vi "Zero.vi"(8 "error in (no error)":errorcluster, 11 "Simple Actor in":refnum<class "Simple Actor.lvclass">) -> (0 "error out":errorcluster, 3 "Simple Actor out":refnum<class "Simple Actor.lvclass">)   [LabVIEW 2012, in "Simple Actor.lvclass"]
uses:
  Simple Actor.lvclass
  Simple Actor.lvclass/Simple Actor.ctl
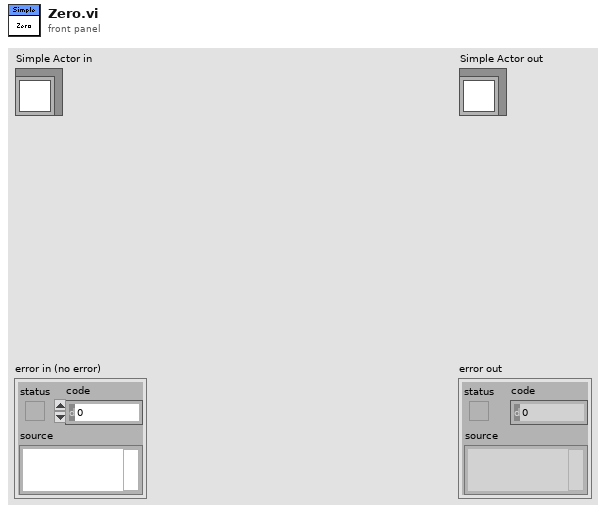
[diagram p1: front panel]
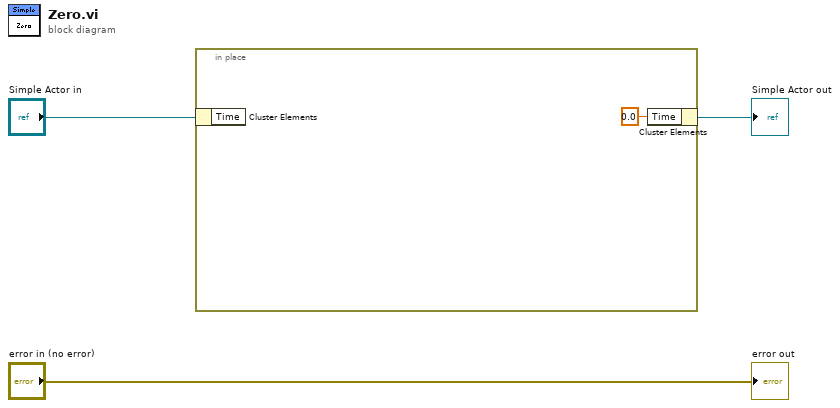
[diagram p0: block diagram]
diagram:
  n1 = in-place {
    n2 = in-place-cluster #1("Simple Actor in") -> ()  [unwired: 1 out]
    n3 = in-place-cluster #1("Time"=0.0) -> (→"Simple Actor out":refnum<class "Simple Actor.lvclass">)
  }
  "error out" <- "error in (no error)"
